vi "Xspress3_Monitor_v3.vi"() -> ()   [LabVIEW 2010]
panel:
  out "DeadTime (%)":dbl[](array[numeric]) format="%#.3f"
  in  "Num of bin":i32=4095
  in  "SaveTime":dbl caption="SaveExposureTime/s"
  in  "save":bool
  in  "Num of ROI":i32=16
  out "Total":dbl caption="TotalExposureTime/s"
  out "Cursor0 Bin":i32=1000
  in  "Num of Ch":i32=8
  out "ROI (cps)":dbl[][](array[numeric]) format="%#.2f"
  in  "Stop":bool
  out "Cursor1 Bin":i32=2000
  out "Graph":cluster{dbl[], dbl[]}[](graph)
  in  "Bin Size":dbl=100.0 format="%#.3f"
  out "ICR (cps)":dbl[](array[numeric]) format="%#.2f"
  in  "Time":dbl=1.0 caption="AcquireTime/s" min=0.1 max=50.0
  in  "ANumber":i32=4096 caption="NumberOfImages" min=1 max=4096 step=1
  in  "Trigger":T1(ring)=enum."Internal"
  # "bin/keV"
  # "2"
  # "3"
  # "4"
  # "5"
  # "6"
  # "7"
  # "8"
  # "9"
  # "10"
  # "11"
  # "12"
  # "13"
  # "14"
  # "15"
  # "16"
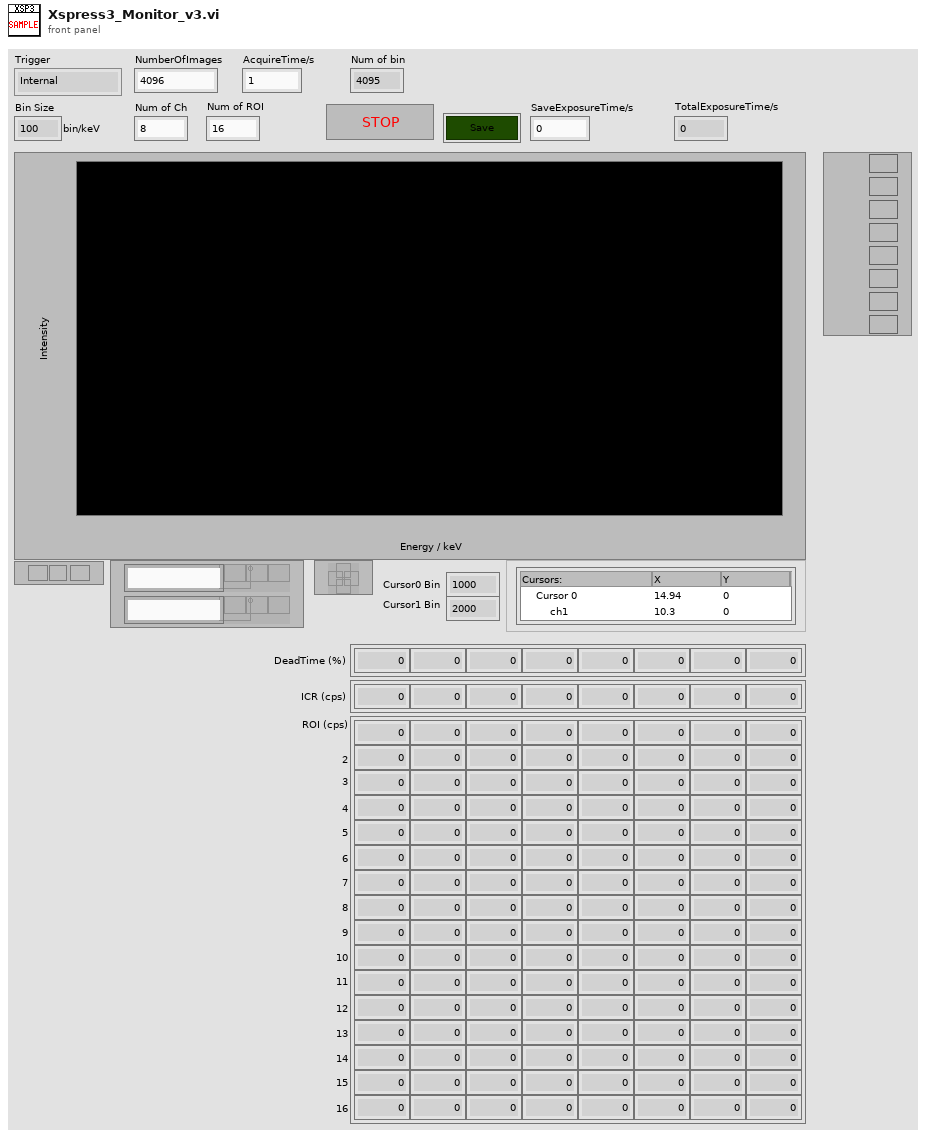
[diagram p1: front panel]
types:
  T1 = enum16{"Software", "Internal", "IDC", "TTL Veto Only", "TTL Both", "LVDS Veto Only", "LVDS Both"}
  T2 = cluster{"MCA":dbl[][], "MCAsum":dbl[][], "ROI/ICRlast":dbl[], "ROI/ICRarray":dbl[][], "DeadTime":dbl[]}
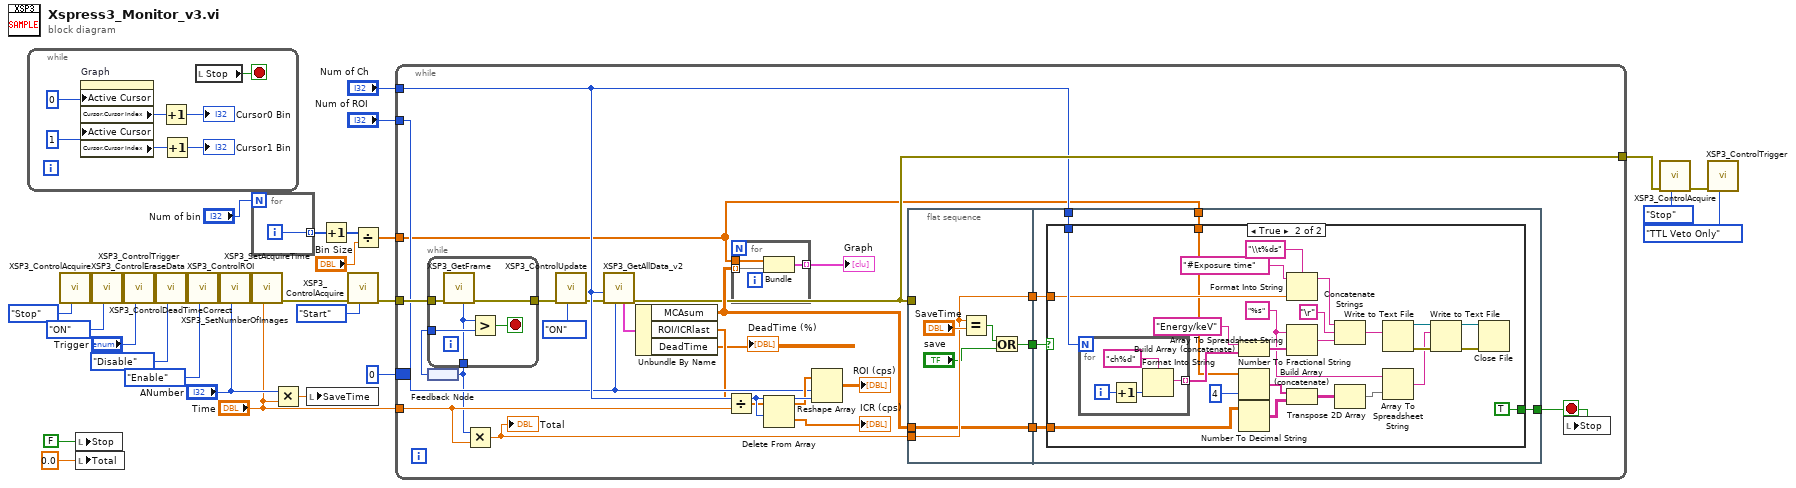
[diagram p0: block diagram]
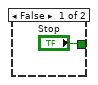
[diagram p2: hidden frame]
diagram:
  n1 = while {
    stop <- w32 stop-if-true
    n2 = property on="Graph" class="XYGraph (strict)"("Active Cursor"=u32 0 ("アクティブカーソル"), "Active Cursor"=u32 1 ("アクティブカーソル")) -> ("Cursor.Cursor Index"=w35:i32, "Cursor.Cursor Index"=w38:i32)  [unwired: 2 in, 2 out]
    n3 = Increment(x=w35) -> (x+1=→"Cursor0 Bin":i32)
    n4 = Increment(x=w38) -> (x+1=→"Cursor1 Bin":i32)
    n5 = local read "Stop"() -> (w32:bool)
  }
  n6 = call "XSP3_ControlAcquire.vi"("Acquire"=enum16{"Stop", "Start"}."Stop") -> ("ErrorOut"=w18:errorcluster)  [unwired: 8 in, 2 out]
  n7 = local write "Stop"(FALSE ("stop")) -> ()
  n8 = local write "Total"(0.0 ("total exposure time")) -> ()
  n9 = call "XSP3_ControlEraseData.vi"("Erase"=enum16{"OFF", "ON"}."ON", "ErrorIn"=w18) -> ("ErrorOut"=w7:errorcluster)  [unwired: 7 in, 2 out]
  n10 = call "XSP3_ControlTrigger.vi"("Trigger"="Trigger", "ErrorIn"=w7) -> ("ErrorOut"=w31:errorcluster)  [unwired: 7 in, 2 out]
  n11 = call "XSP3_ControlDeadTimeCorrect.vi"("DTC"=enum16{"Disable", "Enable"}."Disable", "ErrorIn"=w31) -> ("ErrorOut"=w30:errorcluster)  [unwired: 7 in, 2 out]
  n12 = call "XSP3_ControlROI.vi"("ROIcalc"=enum16{"Disable", "Enable"}."Enable" ("DTC"), "ErrorIn"=w30) -> ("ErrorOut"=w24:errorcluster)  [unwired: 7 in, 2 out]
  n13 = call "XSP3_SetNumberOfImages.vi"("Number"="ANumber", "ErrorIn"=w24) -> ("ErrorOut"=w29:errorcluster)  [unwired: 7 in, 2 out]
  n14 = for {
    N: "Num of bin" -> [_]
    tunnel: [w39] -> w23 mode=indexing
    i -> [w39]
  }
  n15 = call "XSP3_SetAcquireTime.vi"("Time"="Time", "ErrorIn"=w29) -> ("ErrorOut"=w1:errorcluster)  [unwired: 7 in, 2 out]
  n16 = Multiply(x="ANumber", y="Time") -> (x*y=w11:dbl)
  n17 = local write "SaveTime"(w11) -> ()
  n18 = Increment(x=w23) -> (x+1=w9:i32[])
  n19 = call "XSP3_ControlAcquire.vi"("Acquire"=enum16{"Stop", "Start"}."Start" ("Save"), "ErrorIn"=w1) -> ("ErrorOut"=w15:errorcluster)  [unwired: 7 in, 2 out]
  n20 = Divide(x=w9, y="Bin Size") -> (x/y=w8:dbl[])
  n21 = while {
    tunnel: w8 -> [w41]
    tunnel: "Num of Ch" -> [w54]
    tunnel: "Time" -> [w49]
    tunnel: w15 -> [w61]
    tunnel: [w55] -> w10
    tunnel: "Num of ROI" -> [w51]
    border: 0 -> [_]
    stop <- w59 stop-if-true
    n22 = feedback #1() -> (w46:i32)
    n23 = while {
      tunnel: w61 -> [w69]
      tunnel: [w68] -> w43
      tunnel: w46 -> [w72]
      tunnel: [w70] -> w45
      stop <- w71 stop-if-true
      n24 = call "XSP3_GetFrame.vi"("ErrorIn"=w69) -> ("ErrorOut"=w68:errorcluster, "Frame"=w70:i32)  [unwired: 7 in, 2 out]
      n25 = Greater?(x=w70, y=w72) -> (0:w71:bool)
    }
    n26 = feedback-in #1(w45) -> ()
    n27 = Multiply(x=w45, y=w49) -> (x*y=w60:dbl)
    "Total" <- w60
    n28 = call "XSP3_ControlUpdate.vi"("Erase"=enum16{"OFF", "ON"}."ON", "ErrorIn"=w43) -> ("ErrorOut"=w42:errorcluster)  [unwired: 7 in, 2 out]
    n29 = call "XSP3_GetAllData_v2.vi"("NumRoi"=w51, "ErrorIn"=w42, "NumCh"=w54) -> ("ErrorOut"=w55:errorcluster, "Data"=w57:T2)  [unwired: 5 in, 2 out]
    n30 = Unbundle By Name(w57) -> ("MCAsum"=w56:dbl[][], "ROI/ICRlast"=w50:dbl[], "DeadTime"=→"DeadTime (%)":dbl[])
    n31 = Divide(x=w50, y=w49) -> (x/y=w48:dbl[])
    n32 = for {
      tunnel: w56 -> [w66] mode=indexing
      tunnel: w41 -> [w67]
      tunnel: [w65] -> w58 mode=indexing
      n33 = Bundle(w67, "MCAsum"=w66) -> (w65:cluster{dbl[], "MCAsum":dbl[]})  [unwired: 1 in]
    }
    "Graph" <- w58
    n34 = Delete From Array(array=w48, length=w54) -> (deleted portion=→"ICR (cps)":dbl[], array with subset deleted=w52:dbl[])  [unwired: 1 in]
    n35 = Reshape Array(w52, w51, w54) -> (→"ROI (cps)":dbl[][])
    n36 = flat-sequence {
      tunnel: w56 -> [w73]
      tunnel: [w74] -> w64
      tunnel: w60 -> [w77]
      tunnel: [w77] -> w63
      tunnel: [w73] -> w62
      tunnel: w55 -> [_]
      tunnel: w64 -> [w84]
      tunnel: w54 -> [w83]
      tunnel: w63 -> [w82]
      tunnel: w62 -> [w81]
      tunnel: [w80] -> w59
      tunnel: w41 -> [w79]
      frame #0 {
        n37 = Equal?(x=w77, y="SaveTime") -> (x = y?=w76:bool)
        n38 = Or(x=w76, y="save") -> (x .or. y?=w74:bool)
      }
      frame #1 {
        n39 = case shown="True" w84 {
          tunnel: w83 -> [_ w108]
          tunnel: w82 -> [_ w106]
          tunnel: w81 -> [_ w92]
          tunnel: w79 -> [_ w94]
          tunnel: ["Stop" TRUE] -> w80
          frame False {
          }
          frame True {
            w88 = "%s" ("形式文字列")
            n40 = for {
              N: w108 -> [_]
              tunnel: [w111] -> w109 mode=indexing
              i -> [w113]
              n41 = Increment(x=w113) -> (x+1=w112:i32)
              n42 = Format Into String(format string="ch%d", w112) -> (resulting string=w111:string)  [unwired: 2 in, 1 out]
            }
            n43 = Build Array (concatenate)("Energy/keV" ("初期文字列"), w109) -> (w102:string[])
            n44 = Number To Fractional String(number=w94, precision (6)=i16 4 ("精度（6）")) -> (F-format string=w87:string[])  [unwired: 2 in]
            n45 = Number To Decimal String(number=w92) -> (decimal integer string=w91:string[][])  [unwired: 1 in]
            n46 = Format Into String(format string="\\t%ds" ("形式文字列"), initial string="#Exposure time" ("初期文字列"), w106) -> (resulting string=w99:string)  [unwired: 1 in, 1 out]
            n47 = Array To Spreadsheet String(array=w102, 3:w88) -> (spreadsheet string=w101:string)  [unwired: 1 in]
            n48 = Build Array (concatenate)(w87, w91) -> (w90:string[][])
            n49 = Concatenate Strings(w99, "\r", w101) -> (w98:string)
            n50 = Transpose 2D Array(2D array=w90) -> (transposed array=w86:string[][])
            n51 = Write to Text File(text=w98) -> (refnum out=w96:refnum<file>, error out=w97:errorcluster)  [unwired: 3 in, 1 out]
            n52 = Array To Spreadsheet String(array=w86, 3:w88) -> (spreadsheet string=w89:string)  [unwired: 1 in]
            n53 = Write to Text File(file (use dialog)=w96, text=w89, error in=w97) -> (refnum out=w95:refnum<file>, error out=w103:errorcluster)  [unwired: 1 in, 1 out]
            n54 = Close File(refnum=w95, error in=w103) -> ()  [unwired: 2 out]
          }
        }
      }
    }
    n55 = local write "Stop"(w59) -> ()
  }
  n56 = call "XSP3_ControlAcquire.vi"("Acquire"=enum16{"Stop", "Start"}."Stop", "ErrorIn"=w10) -> ("ErrorOut"=w5:errorcluster)  [unwired: 7 in, 2 out]
  n57 = call "XSP3_ControlTrigger.vi"("Trigger"=T1."TTL Veto Only", "ErrorIn"=w5) -> ()  [unwired: 7 in, 3 out]
